vi "DeleteOrder.vi"(11 "buffer.in":u64[](array[numeric])=[0, 0, 0, 0, 0, 0, 0, 0, 0]) -> (3 "OrderBook.Command":T1)   [LabVIEW 2020]
doc: "Cboe PITCH Delete Order (0x29) -> orderbook.command: type DeleteOrder, orderId, nanoseconds, Remove."
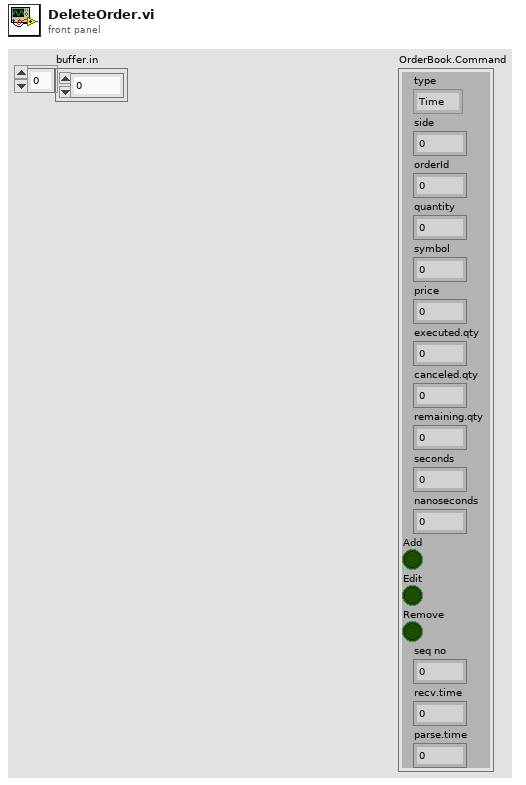
[diagram p1: front panel]
types:
  T1 = cluster{"type":enum8{"Time", "AddOrder", "OrderExecuted", "OrderExecutedAtPrice", "ReduceSize", "ModifyOrder", "DeleteOrder", "Get.Everything", "Get.All.Orders", "Get.Top"}, "side":u8, "orderId ":u64, "quantity":u32, "symbol":u64, "price":u64, "executed.qty":u32, "canceled.qty":u32, "remaining.qty":u32, "seconds":u64, "nanoseconds":u64, "Add":bool, "Edit":bool, "Remove":bool, "seq no":u32, "recv.time":u64, "parse.time":u64}
  T2 = enum8{"Time", "AddOrder", "OrderExecuted", "OrderExecutedAtPrice", "ReduceSize", "ModifyOrder", "DeleteOrder", "Get.Everything", "Get.All.Orders", "Get.Top"}
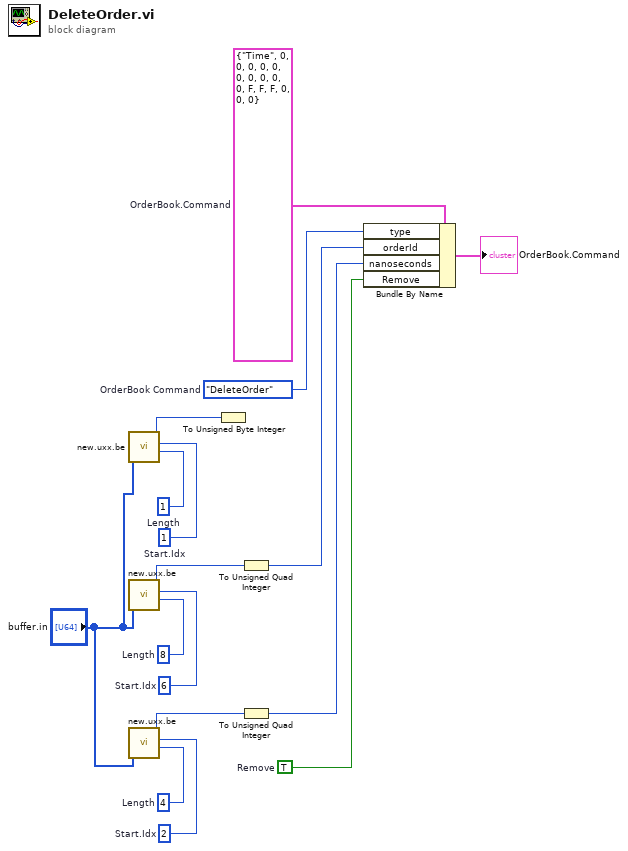
[diagram p0: block diagram]
diagram:
  w8 = u8 8  # Length
  w9 = u8 6  # Start.Idx
  w12 = u8 4  # Length
  w13 = u8 2  # Start.Idx
  w15 = u8 1  # Length
  w16 = u8 1  # Start.Idx
  w3 = TRUE  # Remove
  w6 = T2."DeleteOrder"  # OrderBook Command
  w2 = T1 {"type"=enum."Time", "side"=0, "orderId "=0, "quantity"=0, "symbol"=0, "price"=0, "executed.qty"=0, "canceled.qty"=0, "remaining.qty"=0, "seconds"=0, "nanoseconds"=0, "Add"=FALSE, "Edit"=FALSE, "Remove"=FALSE, "seq no"=0, "recv.time"=0, "parse.time"=0}  # OrderBook.Command
  n1 = call "new.uxx.be.vi"("buffer (U64)"="buffer.in", "Start.Idx"=w16, "Length"=w15) -> ("Out.Value U64"=w14:u64)  [unwired: 7 in]
  n2 = call "new.uxx.be.vi"("buffer (U64)"="buffer.in", "Start.Idx"=w9, "Length"=w8) -> ("Out.Value U64"=w7:u64)  [unwired: 7 in]
  n3 = call "new.uxx.be.vi"("buffer (U64)"="buffer.in", "Start.Idx"=w13, "Length"=w12) -> ("Out.Value U64"=w11:u64)  [unwired: 7 in]
  n4 = To Unsigned Byte Integer(number=w14) -> ()  [unwired: 1 out]
  n5 = To Unsigned Quad Integer(1:w7) -> (0:w5:u64)
  n6 = To Unsigned Quad Integer(1:w11) -> (0:w4:u64)
  n7 = Bundle By Name(cluster=w2, "type"=w6, "orderId"=w5, "nanoseconds"=w4, "Remove"=w3) -> (→"OrderBook.Command":T1)
